vi "Close.vi"(8 "error in (no error)":errorcluster, 11 "CFG Semaphore in":refnum<class "CFG Semaphore.lvclass">) -> (0 "error out":errorcluster, 3 "CFG Semaphore out":refnum<class "CFG Semaphore.lvclass">)   [LabVIEW 2023, in "HAL GOOP4.lvlib" / "CFG Semaphore.lvclass"]
uses:
  CFG Semaphore.lvclass
  CFG Semaphore.lvclass/CFG Semaphore.ctl
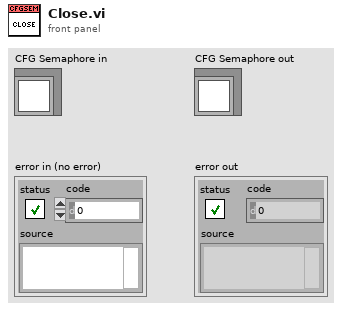
[diagram p1: front panel]
types:
  T1 = typedef "Semaphore RefNum" = refnum<k1>
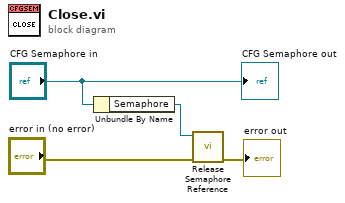
[diagram p0: block diagram]
diagram:
  n1 = Unbundle By Name("CFG Semaphore in") -> ("Semaphore"=w1:T1)
  n2 = call <vilib>:"Release Semaphore Reference.vi"("error in (no error)"="error in (no error)", "semaphore"=w1) -> ("error out"=→"error out":errorcluster)  [unwired: 8 in, 1 out]
  "CFG Semaphore out" <- "CFG Semaphore in"
